vi "_PC_Pub_Move_Window_Horizontally.vi"(1 "HideBtn Ref":refnum<vi>, 2 "Check Bool":bool, 3 "Table Ref":refnum<vi>) -> ()   [LabVIEW 2016]
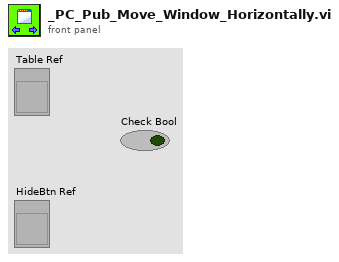
[diagram p1: front panel]
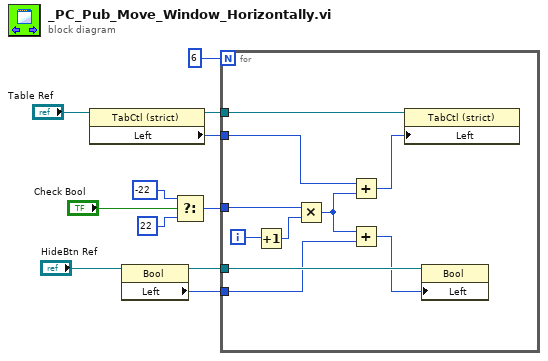
[diagram p0: block diagram]
diagram:
  n1 = property class="TabCtl (strict)"(reference="Table Ref") -> (reference out=w7:refnum<vi>, "Left"=w6:i32)  [unwired: 1 in, 1 out]
  n2 = property class="Bool"(reference="HideBtn Ref") -> (reference out=w4:refnum<vi>, "Left"=w3:i32)  [unwired: 1 in, 1 out]
  n3 = Select(t=-22 ("Left"), s="Check Bool", f=22 ("Left")) -> (s? t:f=w2:i32)
  n4 = for {
    N: 6 -> [_]
    tunnel: w7 -> [w21]
    tunnel: w4 -> [w18]
    tunnel: w2 -> [w14]
    tunnel: w3 -> [w16]
    tunnel: w6 -> [w20]
    i -> [w15]
    n5 = Increment(x=w15) -> (x+1=w13:i32)
    n6 = Multiply(x=w14, y=w13) -> (x*y=w12:i32)
    n7 = Add(x=w20, y=w12) -> (x+y=w19:i32)
    n8 = Add(x=w12, y=w16) -> (x+y=w17:i32)
    n9 = property class="TabCtl (strict)"(reference=w21, "Left"=w19) -> ()  [unwired: 1 in, 2 out]
    n10 = property class="Bool"(reference=w18, "Left"=w17) -> ()  [unwired: 1 in, 2 out]
  }
